vi "GetData.vi"(7 "LabVIEW Web Service Request":refnum<class "Web Request.lvclass">) -> ()   [LabVIEW 2017]
doc: "GetData GET method returns JSON string with last data collected during acquisition."
uses:
  <vilib>/wsapi/Web Request.lvclass
panel:
  # "Use the Web Service Request input terminal to call the VIs on the Web Services palette. Do not remove it from the connector pane unless you don't need access to the palette."
  # "Each additional control wired to the connector pane will be available as an input in the URL. To include an indicator in terminal-mode output (the default setting), it must also be wired to the connector pane."
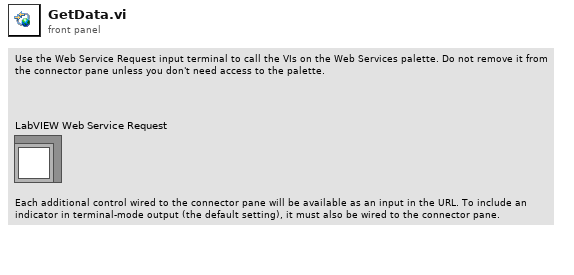
[diagram p1: front panel]
types:
  T1 = cluster{"TemperatureData":dbl, "DIData":bool[], "VRMSData":dbl, "FreqData":dbl}
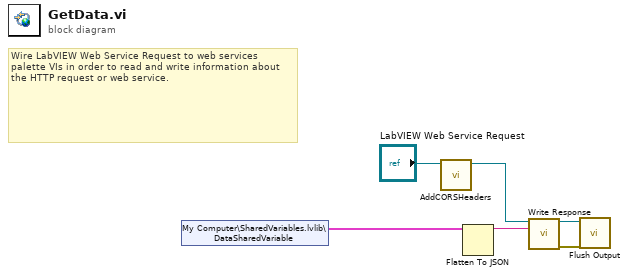
[diagram p0: block diagram]
diagram:
  # "Wire LabVIEW Web Service Request to web services palette VIs in order to read and write information about the HTTP request or web service."
  n1 = shared-variable "My Computer\\SharedVariables.lvlib\\DataSharedVariable"() -> (w1:T1)  [unwired: 1 in, 1 out]
  n2 = call "AddCORSHeaders.vi"("Web Request in"="LabVIEW Web Service Request") -> ("Web Request out"=w2:refnum<class "Web Request.lvclass">)  [unwired: 10 in]
  n3 = Flatten To JSON(anything=w1) -> (JSON string=w6:string)  [unwired: 2 in, 1 out]
  n4 = call <vilib>:"Write Response.vi"("LabVIEW Web Service Request"=w2, "response string"=w6) -> ("LabVIEW Web Service Request out"=w4:refnum<class "Web Request.lvclass">, "error out"=w5:errorcluster)  [unwired: 12 in]
  n5 = call <vilib>:"Flush Output.vi"("LabVIEW Web Service Request"=w4, "error in (no error)"=w5) -> ()  [unwired: 12 in, 2 out]
